vi "Config File Reader (VI Ref).vi"(4 "Parent Label":string, 5 "Parent Class":string, 6 "Close Config File? (T)":bool=TRUE, 7 "This VI":refnum<vi>, 11 "Config File Path":path=path "C:/Users/guillaume/Desktop") -> (3 "Ref Config File Out":T1)   [LabVIEW 2009]
uses:
  <vilib>/Utility/config.llb/Config Data RefNum.ctl
  <vilib>/Utility/config.llb/NI_LVConfig.lvlib
panel:
  # "Guillaume Plateau - Dec. 9, 2009\nyguig2@yahoo.fr - Version 3.0"
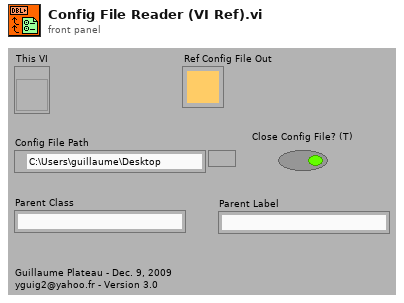
[diagram p1: front panel]
types:
  T1 = typedef "NI_LVConfig.lvlib/Config Data RefNum.ctl" = refnum<k1>
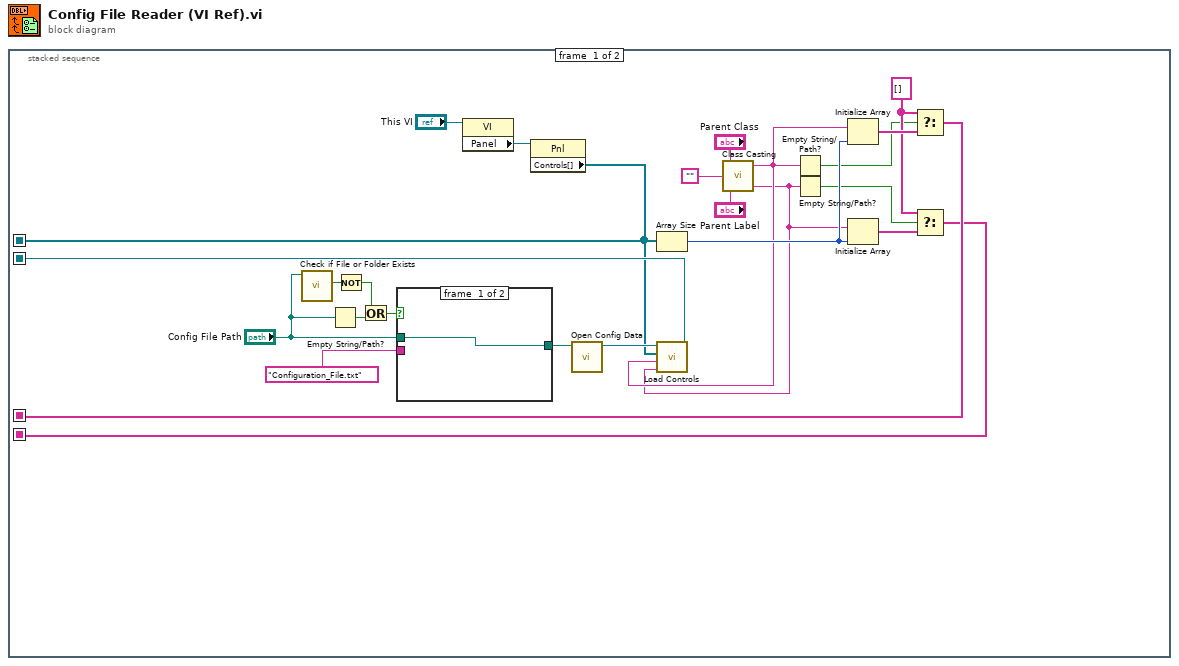
[diagram p0: block diagram]
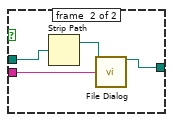
[diagram p2: hidden frame]
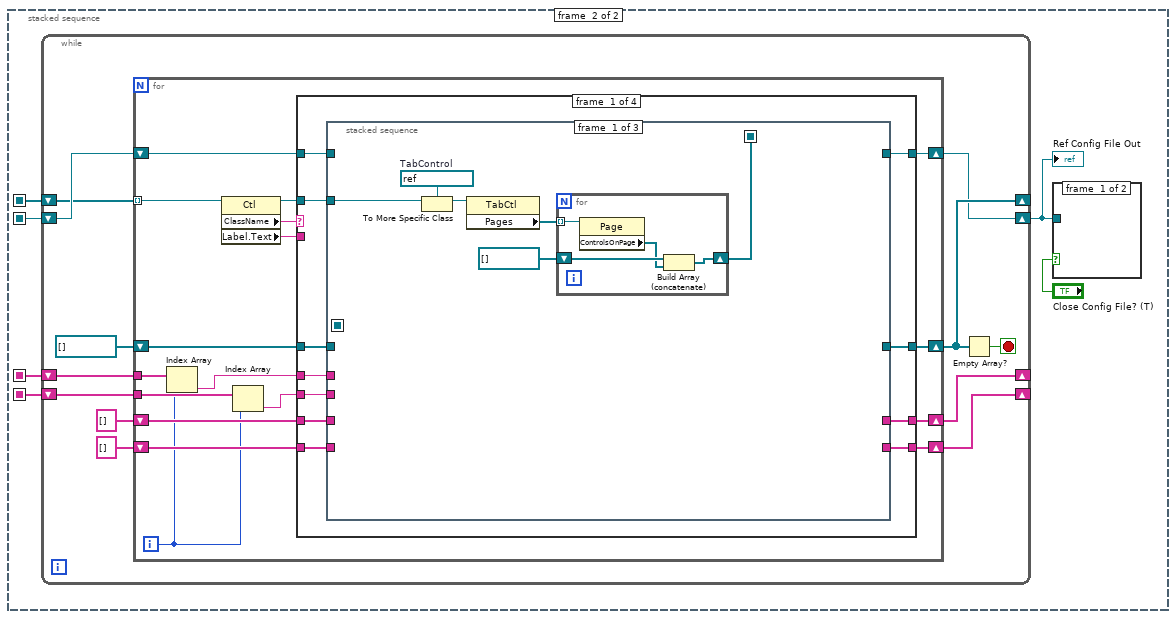
[diagram p3: hidden frame]
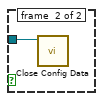
[diagram p4: hidden frame]
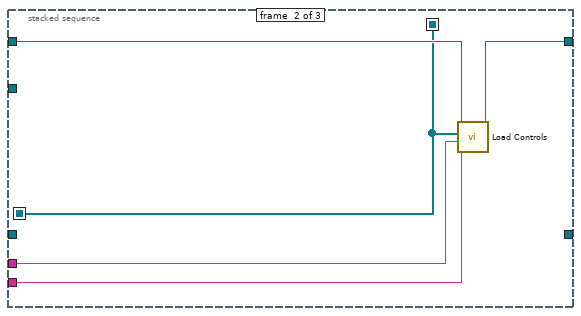
[diagram p5: hidden frame]
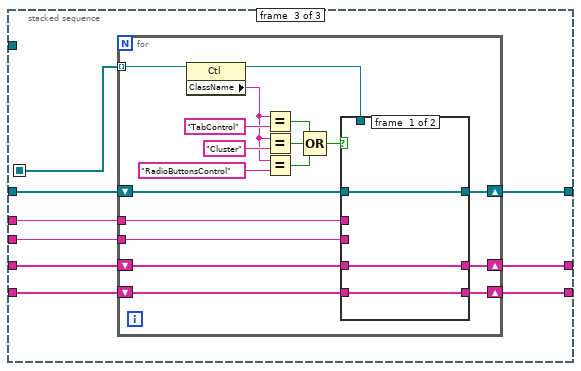
[diagram p6: hidden frame]
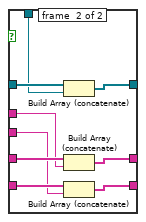
[diagram p7: hidden frame]
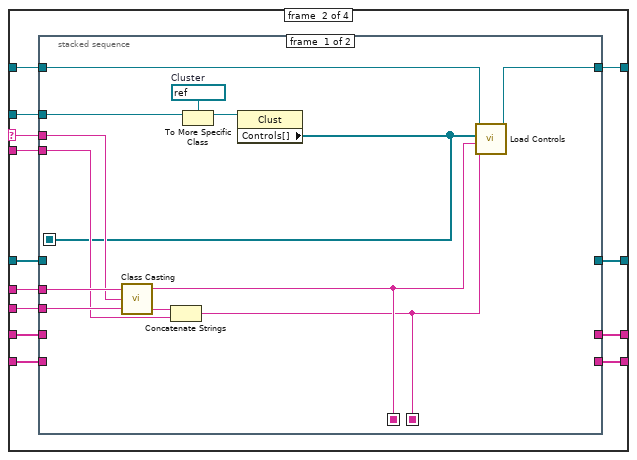
[diagram p8: hidden frame]
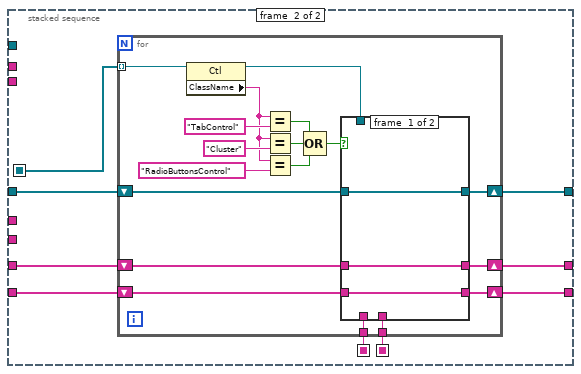
[diagram p9: hidden frame]
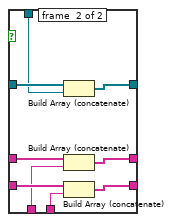
[diagram p10: hidden frame]
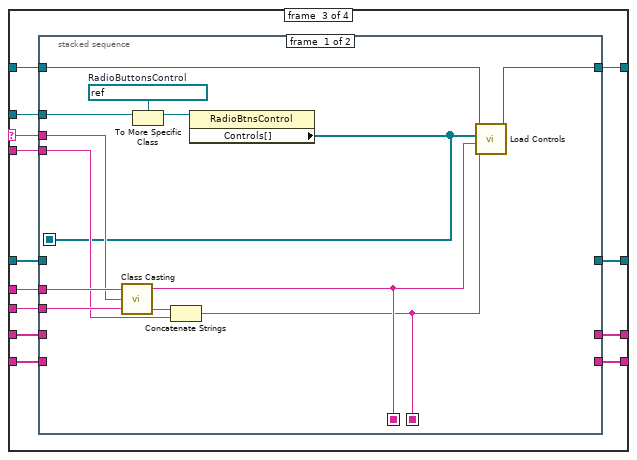
[diagram p11: hidden frame]
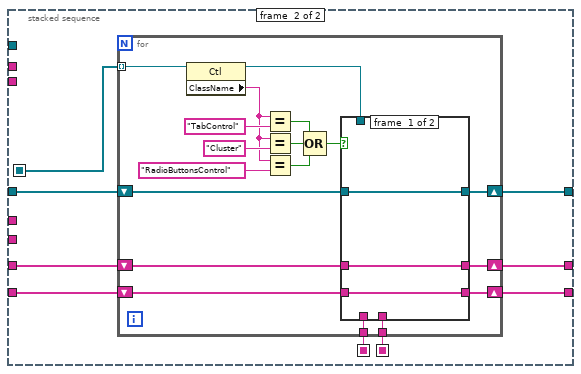
[diagram p12: hidden frame]
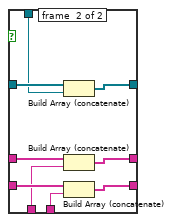
[diagram p13: hidden frame]
diagram:
  n1 = stacked-sequence {
    seq-local: [w1 _] -> [_ w36]
    seq-local: [w17 _] -> [_ w35]
    seq-local: [w9 _] -> [_ w32]
    seq-local: [w8 _] -> [_ w31]
    frame #0 {
      w12 = string[] [] ("t")
      n2 = call <vilib>:"Check if File or Folder Exists.vi"("path"="Config File Path") -> ("file or folder exists?"=w20:bool)  [unwired: 1 in, 9 out]
      n3 = Empty String/Path?(string/path="Config File Path") -> (empty?=w22:bool)
      n4 = Not(x=w20) -> (.not. x?=w18:bool)
      n5 = Or(x=w18, y=w22) -> (x .or. y?=w19:bool)
      n6 = case shown="True" w19 {
        tunnel: "Config File Path" -> [w26 w28]
        tunnel: "Configuration_File.txt" ("name or relative path") -> [_ w30]
        tunnel: [w26 w29] -> w7
        frame #0 {
        }
        frame #1 {
          n7 = Strip Path(path=w28) -> (stripped path=w27:path)  [unwired: 1 out]
          n8 = call "File Dialog"("start path"=w27, "default name"=w30) -> ("selected path"=w29:path)  [unwired: 5 in, 8 out]
        }
      }
      n9 = property class="VI"(reference="This VI") -> ("Panel"=w25:refnum<vi>)  [unwired: 1 in, 2 out]
      n10 = property class="Pnl"(reference=w25) -> ("Controls[]"=w1:refnum<vi>[])  [unwired: 1 in, 2 out]
      n11 = call <vilib>:"Open Config Data.vi"("configuration file path"=w7) -> ("refnum"=w6:T1)  [unwired: 8 in, 2 out]
      n12 = Array Size(array=w1) -> (size(s)=w15:i32)
      n13 = call "Class Casting.vi"("Parent Label"="Parent Label", "Control Class"="", "Parent Class"="Parent Class") -> ("Add-on Label"=w10:string, "Class"=w11:string)  [unwired: 1 out]
      n14 = call "Load Controls.vi"("Parent Label"=w10, "Parent Class"=w11, "Controls[]"=w1, "Ref Config File In"=w6) -> ("Ref Config File Out"=w17:T1)  [unwired: 7 out]
      n15 = Empty String/Path?(string/path=w11) -> (empty?=w5:bool)
      n16 = Empty String/Path?(string/path=w10) -> (empty?=w4:bool)
      n17 = Initialize Array(w11, w15) -> (w14:string[])
      n18 = Initialize Array(w10, w15) -> (w13:string[])
      n19 = Select(t=w12, s=w5, f=w14) -> (s? t:f=w9:string[])
      n20 = Select(t=w12, s=w4, f=w13) -> (s? t:f=w8:string[])
    }
    frame #1 {
      n21 = while {
        shift-right: [w49] -> _
        shift-left: w36 -> [w38]
        shift-right: [w47] -> w33
        shift-left: w35 -> [w48]
        shift-right: [w40] -> _
        shift-left: w32 -> [w44]
        shift-right: [w39] -> _
        shift-left: w31 -> [w43]
        stop <- w45 stop-if-true
        n22 = for {
          tunnel: w38 -> [w59] mode=indexing
          shift-right: [w63] -> w49
          shift-left: refnum<vi>[] [] -> [w64]
          shift-right: [w60] -> w47
          shift-left: w48 -> [w61]
          tunnel: w44 -> [w54]
          tunnel: w43 -> [w53]
          shift-right: [w56] -> w40
          shift-left: string[] [] -> [w58]
          shift-right: [w55] -> w39
          shift-left: string[] [] -> [w57]
          i -> [w52]
          n23 = Index Array(array=w54, index=w52) -> (element=w51:string)
          n24 = property class="Ctl"(reference=w59) -> (reference out=w65:refnum<vi>, "ClassName"=w66:string, "Label.Text"=w62:string)  [unwired: 1 in, 1 out]
          n25 = Index Array(array=w53, index=w52) -> (element=w50:string)
          n26 = case shown="\"TabControl\"" w66 {
            selector: w66 -> [_ w141 w207 _]
            tunnel: w65 -> [w77 w144 w208 _]
            tunnel: w64 -> [w74 w139 w205 w265]
            tunnel: [w73 w138 w199 w265] -> w63
            tunnel: w62 -> [_ w140 w206 _]
            tunnel: w61 -> [w76 w143 w209 w264]
            tunnel: [w75 w142 w200 w264] -> w60
            tunnel: w51 -> [w72 w137 w204 _]
            tunnel: w50 -> [w71 w136 w203 _]
            tunnel: w58 -> [w70 w133 w202 w263]
            tunnel: w57 -> [w69 w132 w201 w262]
            tunnel: [w68 w135 w198 w263] -> w56
            tunnel: [w67 w134 w197 w262] -> w55
            frame #0 {
              n27 = stacked-sequence {
                seq-local: [_ w88 _] -> [_ _ w101]
                seq-local: [w78 _ _] -> [_ w88 _]
                tunnel: w77 -> [w82 _ _]
                tunnel: w76 -> [_ w92 _]
                tunnel: [_ w91 _] -> w75
                tunnel: w74 -> [_ _ w100]
                tunnel: [_ _ w99] -> w73
                tunnel: w72 -> [_ w90 w94]
                tunnel: w71 -> [_ w89 w93]
                tunnel: w70 -> [_ _ w98]
                tunnel: w69 -> [_ _ w97]
                tunnel: [_ _ w96] -> w68
                tunnel: [_ _ w95] -> w67
                frame #0 {
                  w83 = refnum<vi> refnum  # TabControl
                  n28 = To More Specific Class(target class=w83, reference=w82) -> (specific class reference=w81:refnum<vi>)  [unwired: 1 in, 1 out]
                  n29 = property class="TabCtl"(reference=w81) -> ("Pages"=w80:refnum<vi>[])  [unwired: 1 in, 2 out]
                  n30 = for {
                    tunnel: w80 -> [w87] mode=indexing
                    shift-right: [w86] -> w78
                    shift-left: refnum<vi>[] [] -> [w85]
                    n31 = property class="Page"(reference=w87) -> ("ControlsOnPage"=w84:refnum<vi>[])  [unwired: 1 in, 2 out]
                    n32 = Build Array (concatenate)(w85, w84) -> (w86:refnum<vi>[])
                  }
                }
                frame #1 {
                  n33 = call "Load Controls.vi"("Parent Label"=w89, "Parent Class"=w90, "Controls[]"=w88, "Ref Config File In"=w92) -> ("Ref Config File Out"=w91:T1)  [unwired: 7 out]
                }
                frame #2 {
                  n34 = for {
                    tunnel: w101 -> [w119] mode=indexing
                    shift-right: [w109] -> w99
                    shift-left: w100 -> [w110]
                    shift-right: [w105] -> w96
                    shift-left: w98 -> [w108]
                    shift-right: [w104] -> w95
                    shift-left: w97 -> [w107]
                    tunnel: w94 -> [w103]
                    tunnel: w93 -> [w102]
                    n35 = property class="Ctl"(reference=w119) -> (reference out=w106:refnum<vi>, "ClassName"=w112:string)  [unwired: 1 in, 1 out]
                    n36 = Equal?(x=w112, y="TabControl") -> (x = y?=w115:bool)
                    n37 = Equal?(x=w112, y="Cluster") -> (x = y?=w114:bool)
                    n38 = Equal?(x=w112, y="RadioButtonsControl") -> (x = y?=w113:bool)
                    n39 = Compound Arithmetic op=OR(w115, w114, w113) -> (w111:bool)
                    n40 = case shown="True" w111 {
                      tunnel: w110 -> [w122 w131]
                      tunnel: w106 -> [_ w127]
                      tunnel: [w122 w130] -> w109
                      tunnel: w108 -> [w121 w129]
                      tunnel: w107 -> [w120 w128]
                      tunnel: [w121 w126] -> w105
                      tunnel: [w120 w125] -> w104
                      tunnel: w103 -> [_ w124]
                      tunnel: w102 -> [_ w123]
                      frame #0 {
                      }
                      frame #1 {
                        n41 = Build Array (concatenate)(w131, w127) -> (w130:refnum<vi>[])
                        n42 = Build Array (concatenate)(w129, w124) -> (w126:string[])
                        n43 = Build Array (concatenate)(w128, w123) -> (w125:string[])
                      }
                    }
                  }
                }
              }
            }
            frame #1 {
              n44 = stacked-sequence {
                seq-local: [w145 _] -> [_ w166]
                seq-local: [w147 _] -> [_ w159]
                seq-local: [w146 _] -> [_ w158]
                tunnel: w144 -> [w155 _]
                tunnel: w139 -> [_ w160]
                tunnel: [_ w165] -> w138
                tunnel: w143 -> [w154 _]
                tunnel: [w153 _] -> w142
                tunnel: w141 -> [w150 _]
                tunnel: w140 -> [w148 _]
                tunnel: w137 -> [w152 _]
                tunnel: w136 -> [w151 _]
                tunnel: [_ w164] -> w135
                tunnel: [_ w163] -> w134
                tunnel: w133 -> [_ w162]
                tunnel: w132 -> [_ w161]
                frame #0 {
                  w157 = refnum<vi> refnum  # Cluster
                  n45 = call "Class Casting.vi"("Parent Label"=w151, "Control Class"=w150, "Parent Class"=w152) -> ("Add-on Label"=w149:string, "Class"=w147:string)  [unwired: 1 out]
                  n46 = Concatenate Strings(w149, w148) -> (w146:string)
                  n47 = To More Specific Class(target class=w157, reference=w155) -> (specific class reference=w156:refnum<vi>)  [unwired: 1 in, 1 out]
                  n48 = property class="Clust"(reference=w156) -> ("Controls[]"=w145:refnum<vi>[])  [unwired: 1 in, 2 out]
                  n49 = call "Load Controls.vi"("Parent Label"=w146, "Parent Class"=w147, "Controls[]"=w145, "Ref Config File In"=w154) -> ("Ref Config File Out"=w153:T1)  [unwired: 7 out]
                }
                frame #1 {
                  n50 = for {
                    tunnel: w166 -> [w184] mode=indexing
                    shift-right: [w174] -> w165
                    shift-left: w160 -> [w175]
                    shift-right: [w170] -> w164
                    shift-left: w162 -> [w173]
                    shift-right: [w169] -> w163
                    shift-left: w161 -> [w172]
                    tunnel: w159 -> [w168]
                    tunnel: w158 -> [w167]
                    n51 = property class="Ctl"(reference=w184) -> (reference out=w171:refnum<vi>, "ClassName"=w177:string)  [unwired: 1 in, 1 out]
                    n52 = Equal?(x=w177, y="TabControl") -> (x = y?=w180:bool)
                    n53 = Equal?(x=w177, y="Cluster") -> (x = y?=w179:bool)
                    n54 = Equal?(x=w177, y="RadioButtonsControl") -> (x = y?=w178:bool)
                    n55 = Compound Arithmetic op=OR(w180, w179, w178) -> (w176:bool)
                    n56 = case shown="True" w176 {
                      tunnel: w175 -> [w187 w196]
                      tunnel: w171 -> [_ w192]
                      tunnel: [w187 w195] -> w174
                      tunnel: w173 -> [w186 w194]
                      tunnel: w172 -> [w185 w193]
                      tunnel: [w186 w191] -> w170
                      tunnel: [w185 w190] -> w169
                      tunnel: w168 -> [_ w189]
                      tunnel: w167 -> [_ w188]
                      frame #0 {
                      }
                      frame #1 {
                        n57 = Build Array (concatenate)(w196, w192) -> (w195:refnum<vi>[])
                        n58 = Build Array (concatenate)(w194, w189) -> (w191:string[])
                        n59 = Build Array (concatenate)(w193, w188) -> (w190:string[])
                      }
                    }
                  }
                }
              }
            }
            frame #2 {
              n60 = stacked-sequence {
                seq-local: [w210 _] -> [_ w231]
                seq-local: [w215 _] -> [_ w224]
                seq-local: [w214 _] -> [_ w223]
                tunnel: w208 -> [w211 _]
                tunnel: w205 -> [_ w225]
                tunnel: [_ w230] -> w199
                tunnel: w209 -> [w222 _]
                tunnel: [w221 _] -> w200
                tunnel: w207 -> [w218 _]
                tunnel: w206 -> [w216 _]
                tunnel: w204 -> [w220 _]
                tunnel: w203 -> [w219 _]
                tunnel: [_ w229] -> w198
                tunnel: [_ w228] -> w197
                tunnel: w202 -> [_ w227]
                tunnel: w201 -> [_ w226]
                frame #0 {
                  w213 = refnum<vi> refnum  # RadioButtonsControl
                  n61 = call "Class Casting.vi"("Parent Label"=w219, "Control Class"=w218, "Parent Class"=w220) -> ("Add-on Label"=w217:string, "Class"=w215:string)  [unwired: 1 out]
                  n62 = To More Specific Class(target class=w213, reference=w211) -> (specific class reference=w212:refnum<vi>)  [unwired: 1 in, 1 out]
                  n63 = Concatenate Strings(w217, w216) -> (w214:string)
                  n64 = property class="RadioBtnsControl"(reference=w212) -> ("Controls[]"=w210:refnum<vi>[])  [unwired: 1 in, 2 out]
                  n65 = call "Load Controls.vi"("Parent Label"=w214, "Parent Class"=w215, "Controls[]"=w210, "Ref Config File In"=w222) -> ("Ref Config File Out"=w221:T1)  [unwired: 7 out]
                }
                frame #1 {
                  n66 = for {
                    tunnel: w231 -> [w249] mode=indexing
                    shift-right: [w239] -> w230
                    shift-left: w225 -> [w240]
                    shift-right: [w235] -> w229
                    shift-left: w227 -> [w238]
                    shift-right: [w234] -> w228
                    shift-left: w226 -> [w237]
                    tunnel: w224 -> [w233]
                    tunnel: w223 -> [w232]
                    n67 = property class="Ctl"(reference=w249) -> (reference out=w236:refnum<vi>, "ClassName"=w242:string)  [unwired: 1 in, 1 out]
                    n68 = Equal?(x=w242, y="TabControl") -> (x = y?=w245:bool)
                    n69 = Equal?(x=w242, y="Cluster") -> (x = y?=w244:bool)
                    n70 = Equal?(x=w242, y="RadioButtonsControl") -> (x = y?=w243:bool)
                    n71 = Compound Arithmetic op=OR(w245, w244, w243) -> (w241:bool)
                    n72 = case shown="True" w241 {
                      tunnel: w240 -> [w252 w261]
                      tunnel: w236 -> [_ w257]
                      tunnel: [w252 w260] -> w239
                      tunnel: w238 -> [w251 w259]
                      tunnel: w237 -> [w250 w258]
                      tunnel: [w251 w256] -> w235
                      tunnel: [w250 w255] -> w234
                      tunnel: w233 -> [_ w254]
                      tunnel: w232 -> [_ w253]
                      frame #0 {
                      }
                      frame #1 {
                        n73 = Build Array (concatenate)(w261, w257) -> (w260:refnum<vi>[])
                        n74 = Build Array (concatenate)(w259, w254) -> (w256:string[])
                        n75 = Build Array (concatenate)(w258, w253) -> (w255:string[])
                      }
                    }
                  }
                }
              }
            }
            frame #3 {
            }
          }
        }
        n76 = Empty Array?(array=w49) -> (empty?=w45:bool)
      }
      "Ref Config File Out" <- w33
      n77 = case shown="True" "Close Config File? (T)" {
        tunnel: w33 -> [_ w37]
        frame #0 {
        }
        frame #1 {
          n78 = call <vilib>:"Close Config Data.vi"("refnum"=w37) -> ()  [unwired: 2 in, 9 out]
        }
      }
    }
  }
